vi "Split Serial Channel Tap Pairs.vi"(0 "serial channel tap pairs":T1[](array[typedef]), 11 "error in (no error)":errorcluster) -> (4 "serial input channels":string[](array[string]), 6 "serial output channels":string[](array[string]), 15 "error out":errorcluster)   [LabVIEW 2023, in "GettingStarted_Tap_148X_Host.lvlib"]
uses:
  GettingStarted_Tap_148X_Host.lvlib
  Types/Serial Channel Tap Pair.ctl
  <instrlib>/FlexRIO/Automotive Vision Utility/v1/Host/Automotive Vision Utility.lvlib
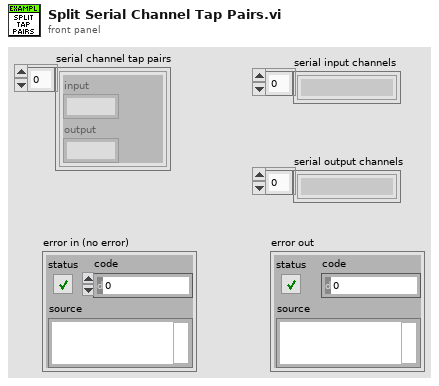
[diagram p1: front panel]
types:
  T1 = typedef "GettingStarted_Tap_148X_Host.lvlib/Serial Channel Tap Pair.ctl" = cluster{"input":string, "output":string}
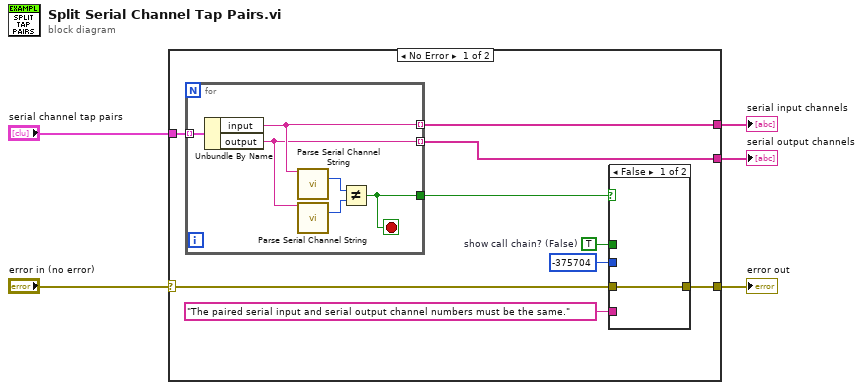
[diagram p0: block diagram]
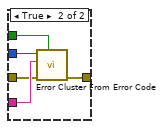
[diagram p2: hidden frame]
diagram:
  n1 = case shown="No Error" "error in (no error)" {
    selector: "error in (no error)" -> [w6 w27]
    tunnel: [w14 _] -> w5
    tunnel: [w13 _] -> w4
    tunnel: "serial channel tap pairs" -> [w12 _]
    tunnel: [w8 w27] -> w1
    frame No Error {
      w10 = TRUE  # show call chain? (False)
      n2 = for {
        tunnel: w12 -> [w26] mode=indexing
        tunnel: [w25] -> w13 mode=indexing
        tunnel: [w24] -> w14 mode=indexing
        tunnel: [w21] -> w7
        stop <- w21 stop-if-true
        n3 = Unbundle By Name(w26) -> ("input"=w25:string, "output"=w24:string)
        n4 = call <instrlib>:"Parse Serial Channel String.vi"("serial channel string"=w25) -> ("channel number"=w23:i32)  [unwired: 13 in, 1 out]
        n5 = call <instrlib>:"Parse Serial Channel String.vi"("serial channel string"=w24) -> ("channel number"=w22:i32)  [unwired: 13 in, 1 out]
        n6 = Not Equal?(x=w23, y=w22) -> (x != y?=w21:bool)
      }
      n7 = case shown="False" w7 {
        tunnel: -375704 ("error code (0)") -> [_ w20]
        tunnel: w10 -> [_ w19]
        tunnel: "The paired serial input and serial output channel numbers must be the same." ("error message (\"\")") -> [_ w18]
        tunnel: [w15 w17] -> w8
        tunnel: w6 -> [w15 w16]
        frame False {
        }
        frame True {
          n8 = call <vilib>:"Error Cluster From Error Code.vi"("show call chain? (False)"=w19, "error in (no error)"=w16, "error message (\"\")"=w18, "error code (0)"=w20) -> ("error out"=w17:errorcluster)  [unwired: 5 in]
        }
      }
    }
    frame Error {
    }
  }
  "serial output channels" <- w5
  "serial input channels" <- w4
  "error out" <- w1
